vi "Rinocloud_HTTP_get_metadata.vi"(8 "error in (no error)":errorcluster, 11 "id":string) -> (0 "error out":errorcluster, 1 "Notes":string, 2 "Tags":string, 3 "Name":string, 4 "Status":T1={"headers"="", "body"="", "ID"="", "Saved"=TRUE}, 5 "metadata (JSON)":string, 7 "JSON Object":variant)   [LabVIEW 2013, in "Rinocloud Library.lvlib"]
uses:
  Rinocloud Library.lvlib
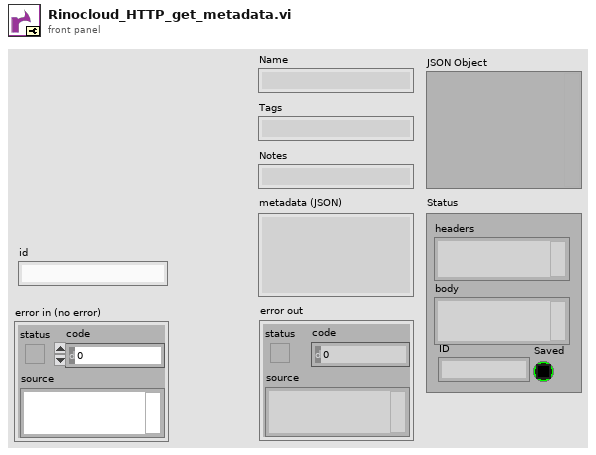
[diagram p1: front panel]
types:
  T1 = cluster{"headers":string, "body":string, "ID":string, "Saved":bool}
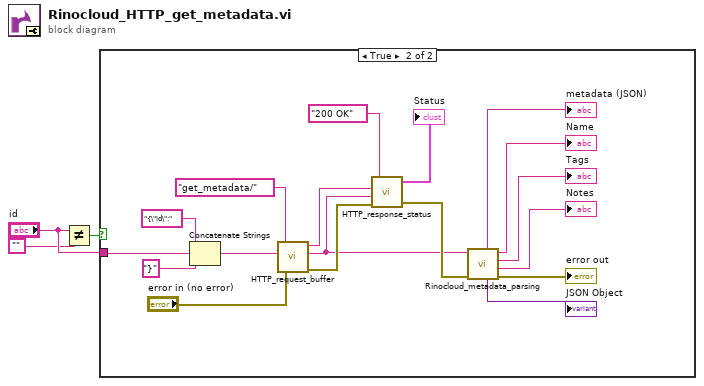
[diagram p0: block diagram]
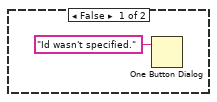
[diagram p2: hidden frame]
diagram:
  n1 = Not Equal?(x="id", y="") -> (x != y?=w3:bool)
  n2 = case shown="True" w3 {
    tunnel: "id" -> [_ w10]
    frame False {
      n3 = One Button Dialog(message="Id wasn't specified.") -> ()  [unwired: 1 in, 1 out]
    }
    frame True {
      n4 = Concatenate Strings("{\"id\":" ("string"), w10, "}" ("string")) -> (w18:string)
      n5 = call "HTTP_request_buffer.vi"("error in (no error)"="error in (no error)", "JSON payload"=w18, "Endpoint"="get_metadata/") -> ("error out"=w20:errorcluster, "body"=w11:string, "headers"=w15:string)  [unwired: 2 in]
      n6 = call "HTTP_response_status.vi"("error in (no error)"=w20, "body"=w11, "headers"=w15, "HTTP status"="200 OK") -> ("error out"=w12:errorcluster, "Status"=→"Status":T1)  [unwired: 1 in]
      n7 = call "Rinocloud_metadata_parsing.vi"("error in (no error)"=w12, "HTTP body"=w11) -> ("error out"=→"error out":errorcluster, "Notes"=→"Notes":string, "Tags"=→"Tags":string, "Name"=→"Name":string, "JSON Object"=→"JSON Object":variant, "metadata (JSON)"=→"metadata (JSON)":string)  [unwired: 4 in]
    }
  }
